vi "InitializePumps.vi"(10 "EquipmentSetup in":refnum<vi>, 11 ".NET Refnum in":refnum<k24>) -> (3 ".NET Refnum out":refnum<k24>)   [LabVIEW 2020]
uses:
  D:/PumpAutomation2/DEMPBot2/PumpAdapter.exe
  PumpAdapter.exe
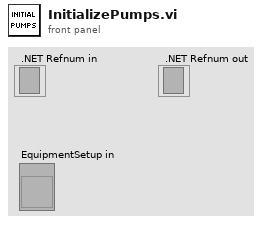
[diagram p1: front panel]
types:
  T1 = typedef "EquipmentDefinition32_1.ctl" = cluster{"VoltageMonitor":tag, "DataDirectory":path, "OverDrawRatio":dbl, "MaxSyringSpeed uL/s":dbl, "Dispense Volume":dbl, "syringeType":i32, "syringeVolume_microliters":i32, "No. of Samples / Loop":i64, "Sampling Rate:":dbl, "Gain (V/nA)":dbl, "Bias channel":tag, "PumpSetups":string[][], "Pump Com Port":string, "CurrentChannels":tag[], "Number Pumps":dbl}
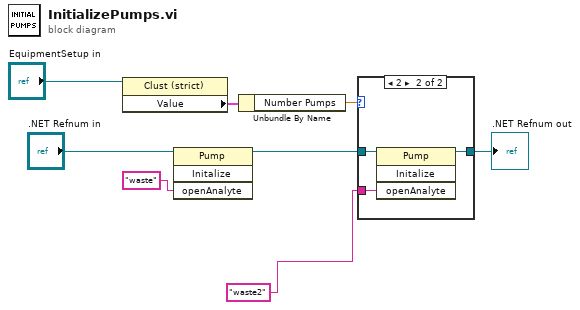
[diagram p0: block diagram]
diagram:
  n1 = property class="Clust (strict)"(reference="EquipmentSetup in") -> ("Value"=w7:T1)  [unwired: 1 in, 2 out]
  n2 = invoke class="Pump" method="Initalize"(reference=".NET Refnum in", "openAnalyte"="waste") -> (reference out=w2:refnum<k24>)  [unwired: 2 in, 3 out]
  n3 = Unbundle By Name(w7) -> ("Number Pumps"=w8:dbl)
  n4 = case shown="2" w8 {
    tunnel: w2 -> [w9 w12]
    tunnel: "waste2" ("openAnalyte") -> [_ w11]
    tunnel: [w9 w10] -> w5
    frame 0, Default {
    }
    frame 2 {
      n5 = invoke class="Pump" method="Initalize"(reference=w12, "openAnalyte"=w11) -> (reference out=w10:refnum<k24>)  [unwired: 2 in, 3 out]
    }
  }
  ".NET Refnum out" <- w5
